vi "BinAdditionSelector.vi"(8 "error in (no error)":errorcluster, 10 "Lower Bounds":dbl[](array[numeric]), 11 "Upper Bounds":dbl[](array[numeric])) -> (0 "error out":errorcluster, 1 "New Highest bound":dbl, 2 "AddLowestBin":bool, 3 "AddHighestBin":bool, 5 "New Lowest bound":dbl)   [LabVIEW 2012, in "Histogram Custom Device.lvlib"]
uses:
  Histogram Custom Device.lvlib
panel:
  in  "Upper Limit":dbl
  in  "Lower Limit":dbl
  out "Lower Limit":dbl
  out "Upper Limit":dbl
  in  "Add Higher Bin?":bool
  in  "Add Lower Bin?":bool
  in  "Done?":bool
  # "Lower Bin"
  # "Higher Bin"
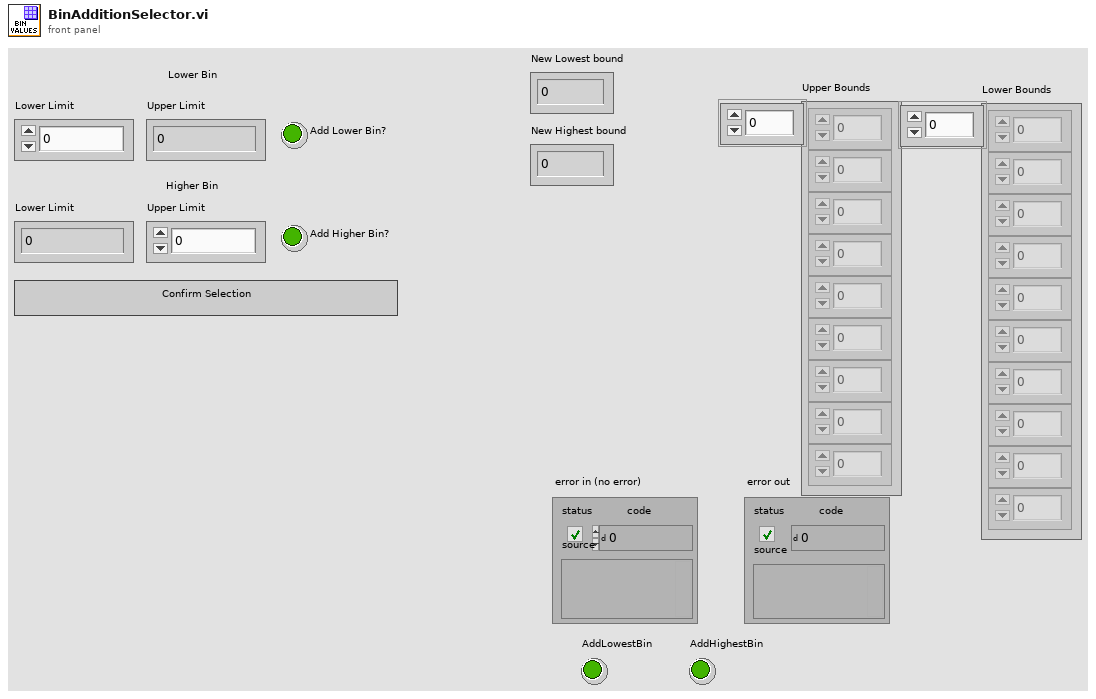
[diagram p1: front panel]
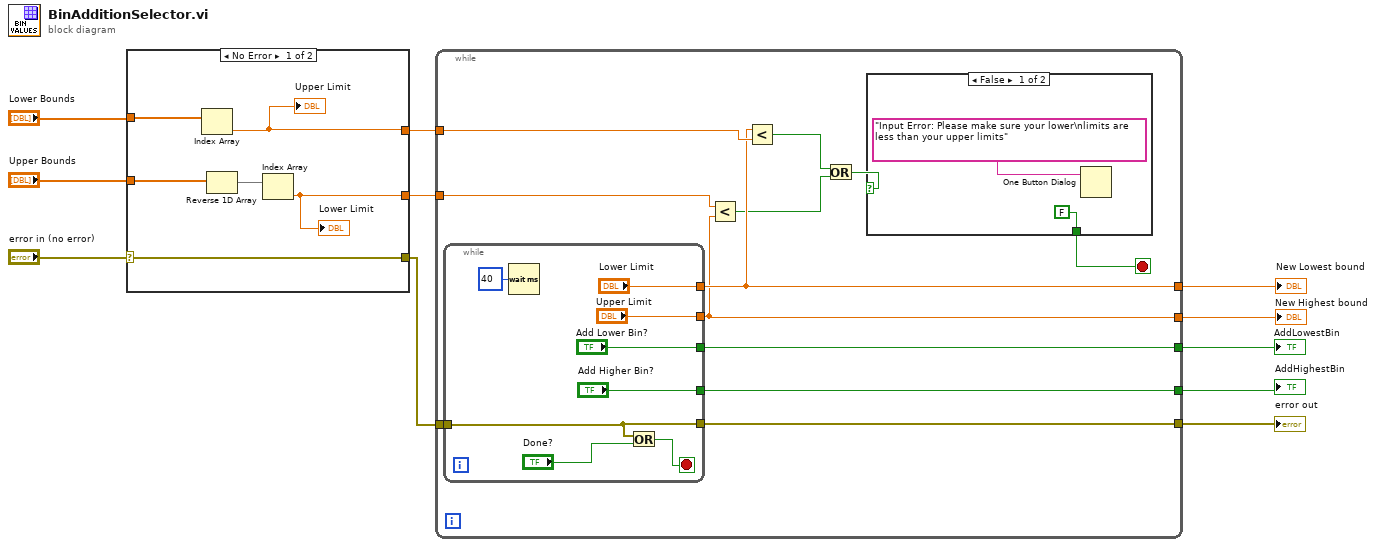
[diagram p0: block diagram]
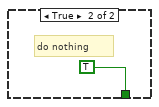
[diagram p2: hidden frame]
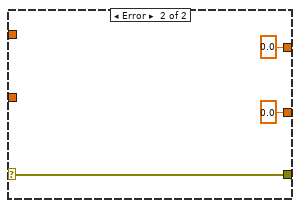
[diagram p3: hidden frame]
diagram:
  n1 = case shown="No Error" "error in (no error)" {
    selector: "error in (no error)" -> [w16 w20]
    tunnel: [w16 w20] -> w10
    tunnel: "Upper Bounds" -> [w15 _]
    tunnel: "Lower Bounds" -> [w14 _]
    tunnel: [w13 0.0 ("String")] -> w4
    tunnel: [w12 0.0 ("String")] -> w2
    frame No Error {
      n2 = Index Array(array=w14) -> (element=w13:dbl)  [unwired: 1 in]
      "Upper Limit" <- w13
      n3 = Reverse 1D Array(array=w15) -> (reversed array=w17:dbl[])
      n4 = Index Array(array=w17) -> (element=w12:dbl)  [unwired: 1 in]
      "Lower Limit" <- w12
    }
    frame Error {
    }
  }
  n5 = while {
    tunnel: w10 -> [w32]
    tunnel: [w31] -> w7
    tunnel: [w30] -> w6
    tunnel: [w29] -> w5
    tunnel: w4 -> [w28]
    tunnel: [w27] -> w3
    tunnel: w2 -> [w26]
    tunnel: [w25] -> w1
    stop <- w21 stop-if-true
    n6 = while {
      tunnel: w32 -> [w40]
      tunnel: [w40] -> w31
      tunnel: ["Add Lower Bin?"] -> w30
      tunnel: ["Add Higher Bin?"] -> w29
      tunnel: ["Lower Limit"] -> w27
      tunnel: ["Upper Limit"] -> w25
      stop <- w42 stop-if-true
      n7 = Wait (ms)(milliseconds to wait=u32 40) -> ()  [unwired: 1 out]
      n8 = Or(x=w40, y="Done?") -> (x .or. y?=w42:bool)
    }
    n9 = Less?(x=w26, y=w25) -> (x < y?=w23:bool)
    n10 = Less?(x=w27, y=w28) -> (x < y?=w24:bool)
    n11 = Or(x=w24, y=w23) -> (x .or. y?=w22:bool)
    n12 = case shown="False" w22 {
      tunnel: [FALSE TRUE] -> w21
      frame False {
        n13 = One Button Dialog(message="Input Error: Please make sure your lower\nlimits are less than your upper limits") -> ()  [unwired: 1 in, 1 out]
      }
      frame True {
        # "do nothing"
      }
    }
  }
  "error out" <- w7
  "AddHighestBin" <- w5
  "AddLowestBin" <- w6
  "New Lowest bound" <- w3
  "New Highest bound" <- w1
